vi "Update LCD.vi"(8 "error in (no error)":errorcluster, 11 "Front Panel Emulator in":refnum<class "Front Panel Emulator.lvclass">) -> (0 "error out":errorcluster)   [LabVIEW 2020, in "Front Panel Emulator.lvlib" / "Front Panel Emulator.lvclass"]
uses:
  Front Panel Emulator.lvclass
  Front Panel Emulator.lvclass/Front Panel Emulator.ctl
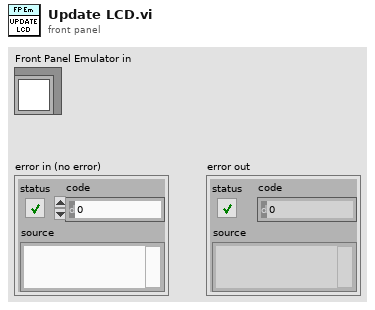
[diagram p1: front panel]
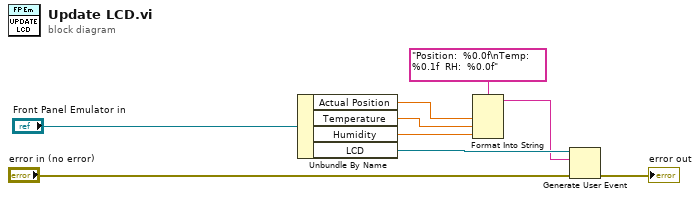
[diagram p0: block diagram]
diagram:
  n1 = Unbundle By Name("Front Panel Emulator in") -> ("Actual Position"=w3:dbl, "Temperature"=w4:dbl, "Humidity"=w5:dbl, "LCD"=w7:refnum<user-event>)
  n2 = Format Into String(format string="Position:  %0.0f\nTemp:  %0.1f  RH:  %0.0f", w3, w4, w5) -> (resulting string=w6:string)  [unwired: 2 in, 1 out]
  n3 = Generate User Event(user event=w7, event data cluster=w6, error in="error in (no error)") -> (error out=→"error out":errorcluster)  [unwired: 1 in, 1 out]
